vi "Configure Waveform (Arbitrary).vi"(0 "VISA resource name":refnum<visa-resource-name>, 1 "Frequency (1000 Hz)":dbl=1000.0 min=1e-06 max=10000000.0, 5 "Arbitrary Waveform Name (\"EXP_RISE\")":string="EXP_RISE", 9 "Gain (1.0 Vpp)":dbl=1.0, 11 "error in (no error)":errorcluster, 12 "DC Offset (0.00 V)":dbl) -> (4 "VISA resource name out":refnum<visa-resource-name>, 15 "error out":errorcluster)   [LabVIEW 2017, in "Keithley 3390.lvlib"]
doc: "Sets the waveform parameters for an arbitrary waveform and makes it the active waveform function. This VI should be called after Create Arbitrary Waveform."
uses:
  Keithley 3390.lvlib
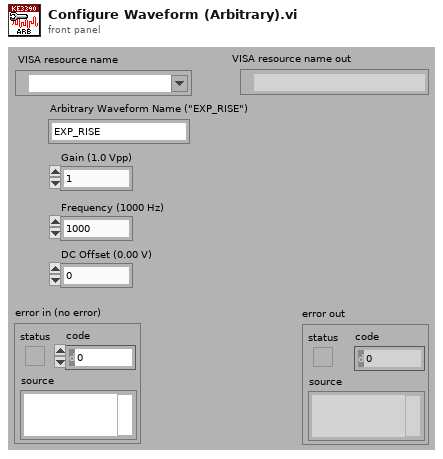
[diagram p1: front panel]
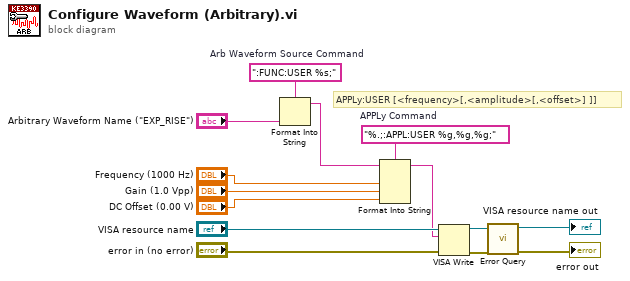
[diagram p0: block diagram]
diagram:
  w7 = ":FUNC:USER %s;"  # Arb Waveform Source Command
  w8 = "%.;:APPL:USER %g,%g,%g;"  # APPLy Command
  # "APPLy:USER [<frequency>[,<amplitude>[,<offset>] ]]"
  n1 = Format Into String(format string=w7, "Arbitrary Waveform Name (\"EXP_RISE\")") -> (resulting string=w2:string)  [unwired: 2 in, 1 out]
  n2 = Format Into String(format string=w8, initial string=w2, "Frequency (1000 Hz)", "Gain (1.0 Vpp)", "DC Offset (0.00 V)") -> (resulting string=w1:string)  [unwired: 1 in, 1 out]
  n3 = VISA Write(VISA resource name="VISA resource name", write buffer=w1, error in (no error)="error in (no error)") -> (VISA resource name out=w14:refnum<visa-resource-name>, error out=w13:errorcluster)  [unwired: 1 out]
  n4 = call "Error Query.vi"("error in (no error)"=w13, "VISA resource name"=w14) -> ("error out"=→"error out":errorcluster, "VISA resource name out"=→"VISA resource name out":refnum<visa-resource-name>)  [unwired: 6 in, 2 out]
